vi "Update Quantity in Inventory.vi"(8 "error in":errorcluster, 11 "Inventory In":T1[](array[typedef])) -> (0 "error out":errorcluster, 2 "Inventory Out  for Undu2":T1[](array[typedef]), 3 "Inventory Out":T1[](array[typedef]))   [LabVIEW 2013]
uses:
  Controls/Display Component Line.ctl
  Controls/Components.ctl
  Controls/Component Sub Type.ctl
  Controls/Add Button.ctl
  Controls/Subtract Button.ctl
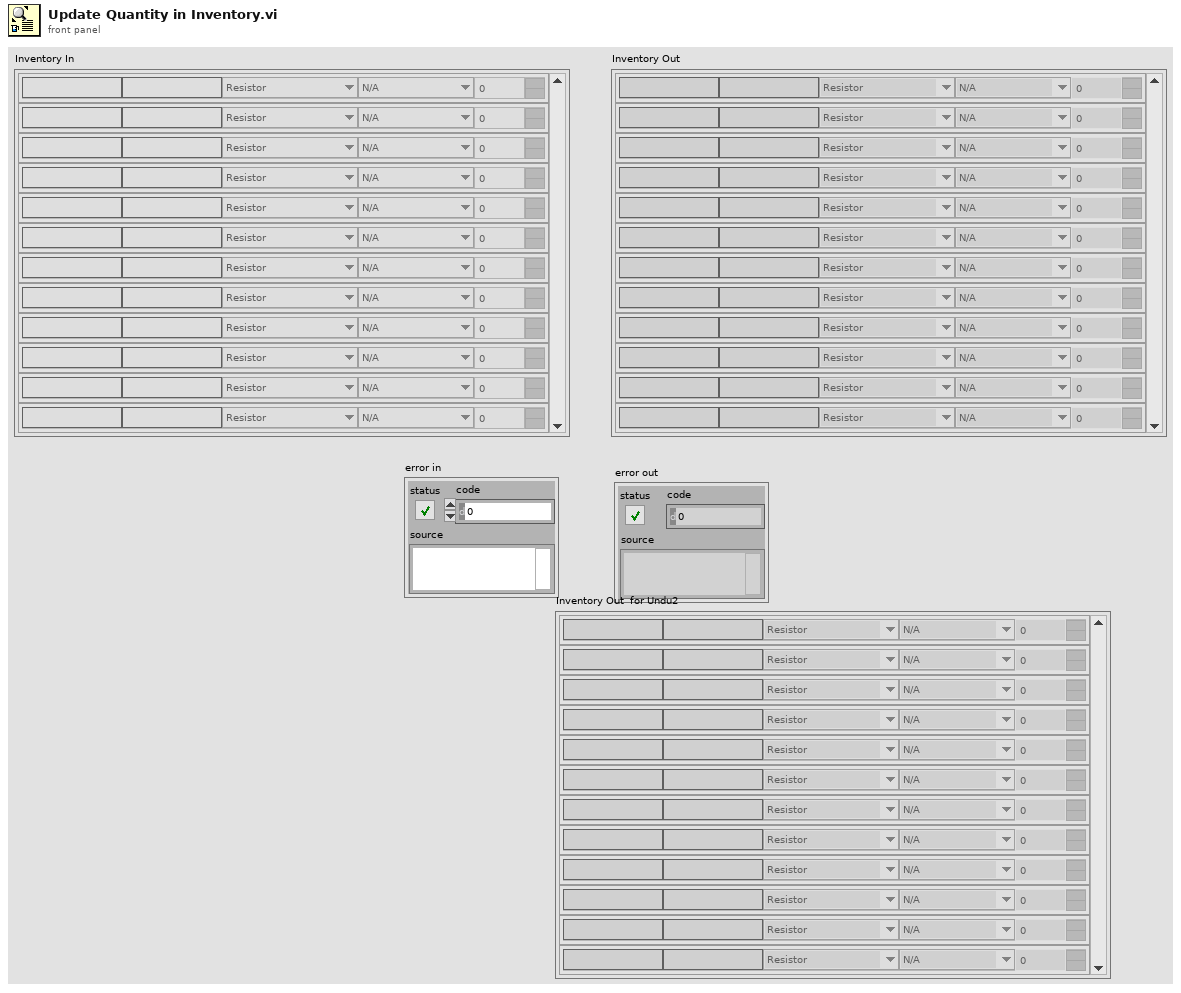
[diagram p1: front panel]
types:
  T1 = typedef "Display Component Line.ctl" = cluster{"Part Number":string, "Code (Value)":string, "Component Type":T2, "Component Subtype":T3, "Quantity":u32, "Add":T4, "Subtract":T5}
  T2 = typedef "Components.ctl" = enum16{"Resistor", "Capacitor", "Diode", "Voltage Regulator"}
  T3 = typedef "Component Sub Type.ctl" = enum16{"N/A", "Ceramic", "Electrolitic", "Zenner", "NPN", "PNP"}
  T4 = typedef "Add Button.ctl" = bool
  T5 = typedef "Subtract Button.ctl" = bool
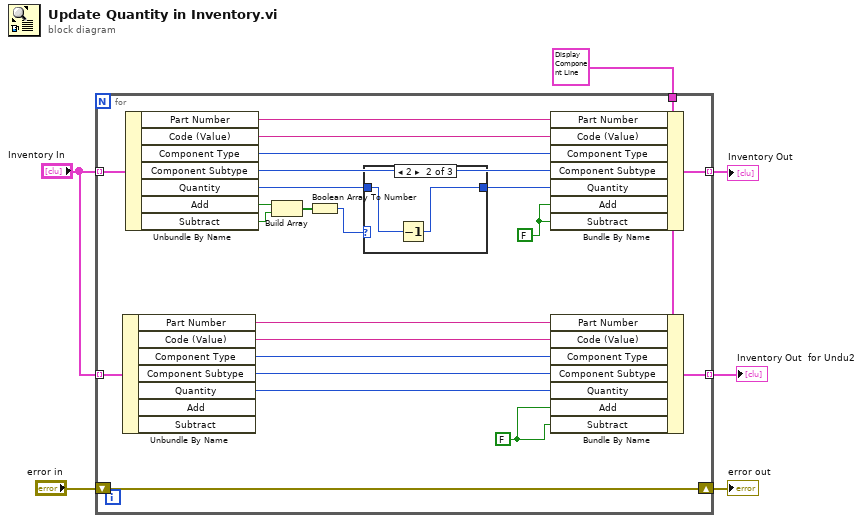
[diagram p0: block diagram]
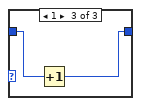
[diagram p3: hidden frame]
diagram:
  n1 = for {
    tunnel: "Inventory In" -> [w29] mode=indexing
    tunnel: [w23] -> w6 mode=indexing
    shift-right: [w22] -> w4
    shift-left: "error in" -> [w22]
    tunnel: T1 {"Part Number"="", "Code (Value)"="102", "Component Type"=enum."Capacitor", "Component Subtype"=enum."Ceramic", "Quantity"=10, "Add"=TRUE, "Subtract"=FALSE} ("Display Components Line") -> [w12]
    tunnel: [w15] -> w2 mode=indexing
    tunnel: "Inventory In" -> [w14] mode=indexing
    w7 = FALSE
    w28 = FALSE
    n2 = Unbundle By Name(w14) -> ("Part Number"=w13:string, "Code (Value)"=w11:string, "Component Type"=w10:T2, "Component Subtype"=w9:T3, "Quantity"=w8:u32)  [unwired: 2 out]
    n3 = Unbundle By Name(w29) -> ("Part Number"=w24:string, "Code (Value)"=w25:string, "Component Type"=w26:T2, "Component Subtype"=w27:T3, "Quantity"=w17:u32, "Add"=w21:T4, "Subtract"=w20:T5)
    n4 = Build Array(w21, w20) -> (w19:T5[])
    n5 = Boolean Array To Number(Boolean array=w19) -> (number=w18:u32)
    n6 = case shown="2" w18 {
      tunnel: w17 -> [w30 w32 w34]
      tunnel: [w30 w31 w33] -> w16
      frame Default {
      }
      frame 2 {
        n7 = Decrement(x=w32) -> (x-1=w31:u32)
      }
      frame 1 {
        n8 = Increment(x=w34) -> (x+1=w33:u32)
      }
    }
    n9 = Bundle By Name(cluster=w12, "Part Number"=w24, "Code (Value)"=w25, "Component Type"=w26, "Component Subtype"=w27, "Quantity"=w16, "Add"=w28, "Subtract"=w28) -> (w23:T1)
    n10 = Bundle By Name(cluster=w12, "Part Number"=w13, "Code (Value)"=w11, "Component Type"=w10, "Component Subtype"=w9, "Quantity"=w8, "Add"=w7, "Subtract"=w7) -> (w15:T1)
  }
  "Inventory Out" <- w6
  "error out" <- w4
  "Inventory Out  for Undu2" <- w2
